vi "2023_day16 (SubVI Append Unvisited Energized Tile to Log).vi"(6 "Next Direction":enum16{"UP", "LEFT", "DOWN", "RIGHT"}(ring), 7 "Next Position (Row,Col)":i32[](array[numeric]), 11 "Beam in":T1) -> (1 "Stop":bool, 3 "Beam out":T1)   [LabVIEW 2021]
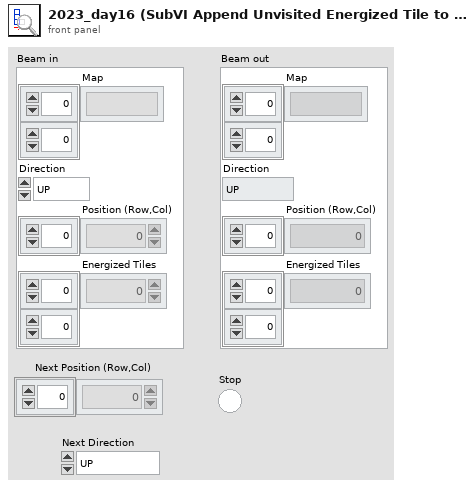
[diagram p1: front panel]
types:
  T1 = cluster{"Map":string[][], "Direction":enum16{"UP", "LEFT", "DOWN", "RIGHT"}, "Position (Row,Col)":i32[], "Energized Tiles":i32[][]}
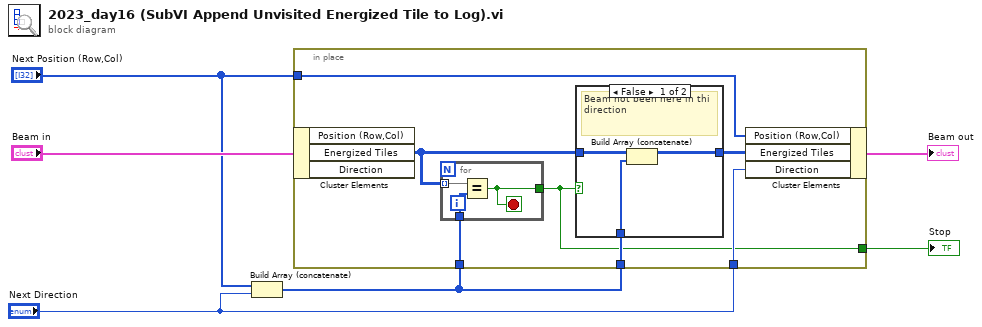
[diagram p0: block diagram]
diagram:
  n1 = Build Array (concatenate)("Next Position (Row,Col)", "Next Direction") -> (w2:i32[])
  n2 = in-place {
    in-place-border: "Next Position (Row,Col)" -> [w13]
    in-place-border: "Next Direction" -> [w12]
    in-place-border: w2 -> [w9]
    in-place-border: w2 -> [w8]
    in-place-border: [w7] -> w1
    n3 = in-place-cluster #1("Beam in") -> ("Energized Tiles"=w11:i32[][])  [unwired: 2 out]
    n4 = for {
      tunnel: w11 -> [w16] mode=indexing
      tunnel: w8 -> [w15]
      tunnel: [w14] -> w7
      stop <- w14 stop-if-true
      n5 = Equal?(x=w16, y=w15) -> (x = y?=w14:bool)
    }
    n6 = case shown="False" w7 {
      tunnel: w11 -> [w19 w20]
      tunnel: [w18 w20] -> w10
      tunnel: w9 -> [w17 _]
      frame False {
        # "Beam not been here in thi direction"
        n7 = Build Array (concatenate)(w19, w17) -> (w18:i32[][])
      }
      frame True {
        # "Stop beam from running in infinite loop"
      }
    }
    n8 = in-place-cluster #1("Position (Row,Col)"=w13, "Energized Tiles"=w10, "Direction"=w12) -> (→"Beam out":T1)
  }
  "Stop" <- w1
